vi "Using Temperature.vi"(10 "Delay Multiplier":dbl(knob)=1.0 min=0.0 max=2.0 step=0.1 scale=0.0..2.0, 11 "Number of Measurements":i32=100) -> (3 "Temperature Chart":dbl(graph))   [LabVIEW 2012]
panel:
  in  "Stop Button":bool
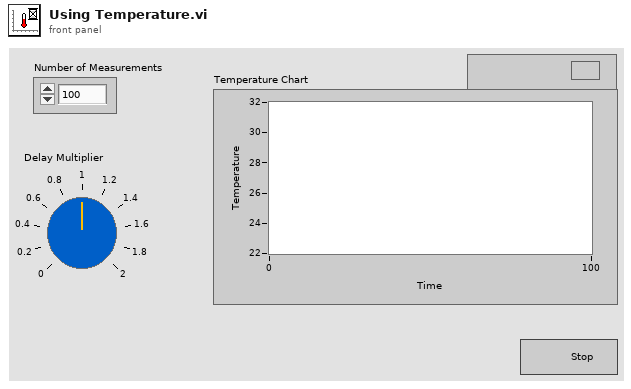
[diagram p1: front panel]
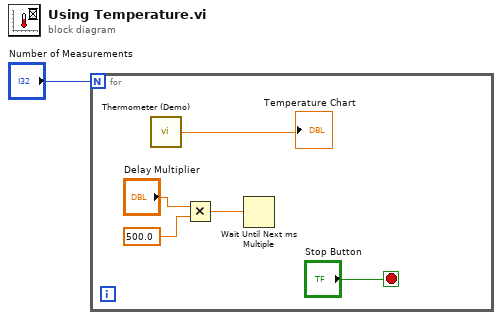
[diagram p0: block diagram]
diagram:
  n1 = for {
    N: "Number of Measurements" -> [_]
    stop <- "Stop Button" stop-if-true
    n2 = call "Thermometer (Demo).vi"() -> ("Temperature Value"=→"Temperature Chart":dbl)  [unwired: 1 in]
    n3 = Multiply(x="Delay Multiplier", y=500.0) -> (x*y=w4:dbl)
    n4 = Wait Until Next ms Multiple(millisecond multiple=w4) -> ()  [unwired: 1 out]
  }
